vi "Get Acquired Data.vi"(8 "error in (no error)":errorcluster, 11 "CCDCamera in":refnum<class "CCDCamera.lvclass">) -> (0 "error out":errorcluster, 3 "CCDCamera out":refnum<class "CCDCamera.lvclass">)   [LabVIEW 2018, in "CCDCamera.lvclass"]
uses:
  CCDCamera.lvclass
  C:/Users/observer/Desktop/SPARC4_ACS/SPARC4_ACS/Simulated_CCD_Camera/Simulated_CCD_Camera.lvclass
  Simulated_CCD_Camera/Simulated_CCD_Camera.lvclass
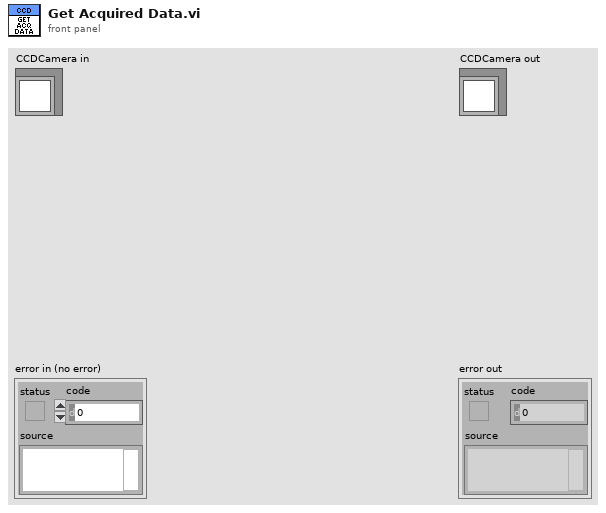
[diagram p1: front panel]
types:
  T1 = cluster{"CUBE_EXPOSURE_TIME":sgl, "CUBES_DONE":u16, "LAST_IMAGE_NAME":string, "DISK_SPACE":u16, "FRAMES_DONE":u16, "CCD_STATUS":string, "CURRENT_TEMPERATURE":i16, "TEMPERATURE_STATUS":string, "FRAME_EXPOSURE_TIME":dbl, "CCD_POWER_STATUS":bool, "SERIAL_NUMBER":u16, "ACQUIRING":bool}
  T2 = cluster{"PREAMP":u16, "READOUT_RATE":u16, "EM_GAIN":u16, "VERTICAL_SHIFT_SPEED":u16, "READ_MODE":u16, "FRAME_TRANSFER":bool, "VERTICAL_CLOCK_VOLTAGE":u16, "ACQUISITION_MODE":u16, "AD_CHANNEL":u16, "EM_MODE":u16, "SHUTTER_TTL":u16, "SHUTTER_OPENING_TIME":u16, "SHUTTER_CLOSING_TIME":u16, "SHUTTER_MODE":u16, "TRIGGER_MODE":u16, "VBIN":u16, "INITIAL_LINE":u16, "INITIAL_COLUMN":u16, "FINAL_LINE":u16, "FINAL_COLUMN":u16, "HBIN":u16}
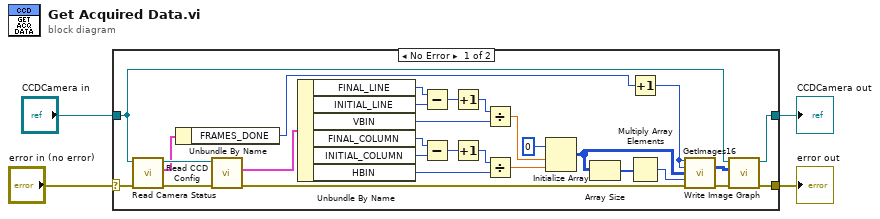
[diagram p0: block diagram]
diagram:
  n1 = case shown="No Error" "error in (no error)" {
    selector: "error in (no error)" -> [w11 w35]
    tunnel: [w22 w35] -> w1
    tunnel: [w21 w34] -> w2
    tunnel: "CCDCamera in" -> [w8 w34]
    frame No Error {
      n2 = call "Read Camera Status.vi"("error in (no error)"=w11, "CCDCamera in"=w8) -> ("error out"=w10:errorcluster, "Camera Status"=w7:T1, "CCDCamera out"=w9:refnum<class "CCDCamera.lvclass">)  [unwired: 7 in]
      n3 = Unbundle By Name(w7) -> ("FRAMES_DONE"=w6:u16)
      n4 = call "Read CCD Config.vi"("error in (no error)"=w10, "CCDCamera in"=w9) -> ("error out"=w13:errorcluster, "CCD Config"=w12:T2)  [unwired: 7 in, 1 out]
      n5 = Unbundle By Name(w12) -> ("FINAL_LINE"=w14:u16, "INITIAL_LINE"=w15:u16, "VBIN"=w16:u16, "FINAL_COLUMN"=w17:u16, "INITIAL_COLUMN"=w18:u16, "HBIN"=w19:u16)
      n6 = Subtract(x=w14, y=w15) -> (x-y=w33:u16)
      n7 = Subtract(x=w17, y=w18) -> (x-y=w32:u16)
      n8 = Increment(x=w33) -> (x+1=w31:u16)
      n9 = Increment(x=w32) -> (x+1=w30:u16)
      n10 = Divide(x=w31, y=w16) -> (x/y=w28:dbl)
      n11 = Divide(x=w30, y=w19) -> (x/y=w27:dbl)
      n12 = Initialize Array(u16 0, w28, w27) -> (w26:u16[][])
      n13 = Array Size(array=w26) -> (size(s)=w25:i32[])
      n14 = Increment(x=w6) -> (x+1=w5:u16)
      n15 = Multiply Array Elements(1:w25) -> (0:w24:i32)
      n16 = call <userlib>:"GetImages16.vi"("first"=w5, "last"=w5, "array"=w26, "size"=w24, "error in (no error)"=w13) -> ("array"=w20:u16[][], "error out"=w23:errorcluster)  [unwired: 6 in, 3 out]
      n17 = call-dynamic "Write Image Graph.vi"("error in (no error)"=w23, "Image Graph"=w20, "CCDCamera in"=w8) -> ("error out"=w22:errorcluster, "CCDCamera out"=w21:refnum<class "CCDCamera.lvclass">)  [unwired: 7 in]
    }
    frame Error {
    }
  }
  "error out" <- w1
  "CCDCamera out" <- w2
